vi "Thrust Allocation().vi"() -> (3 "Thrust Allocation Out":refnum<class "Thrust Allocation.lvclass">)   [LabVIEW 2014, in "Thrust Allocation.lvclass"]
uses:
  Thrust Allocation.lvclass
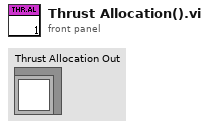
[diagram p1: front panel]
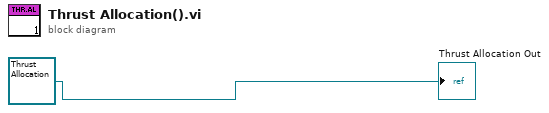
[diagram p0: block diagram]
diagram:
  "Thrust Allocation Out" <- refnum<class "Thrust Allocation.lvclass"> refnum ("Thrust Allocation.lvclass")
